vi "LVRT Serial Init.vi"(6 "stop bits (10: 1 bit)":u16(ring)=10 items=["1 bit"=10, "1.5 bits"=15, "2 bits"=20], 7 "Invert Polarity?":bool, 8 "error in (no error)":errorcluster, 9 "parity (0:none)":u16(ring) items=["None", "Odd", "Even", "Mark", "Space"], 10 "data bits (8)":u16=8 min=5 max=8 step=1, 11 "baud rate (9600)":u32=9600) -> (0 "error out":errorcluster, 3 "FPGA Main Reference Out":refnum<k20>)   [LabVIEW 2009]
uses:
  <vilib>/rvi/interface/nirviMethod/nirviMethod.xnode
  <vilib>/rvi/interface/nirviOpenFPGA/nirviOpenFPGA.xnode
  <vilib>/rvi/interface/nirviReadWriteControl/nirviReadWriteControl.xnode
  FPGA Main.vi
  FPGA Bitfiles/FPGA RS232.lvproj_FPGA Target_FPGA Main.vi.lvbit
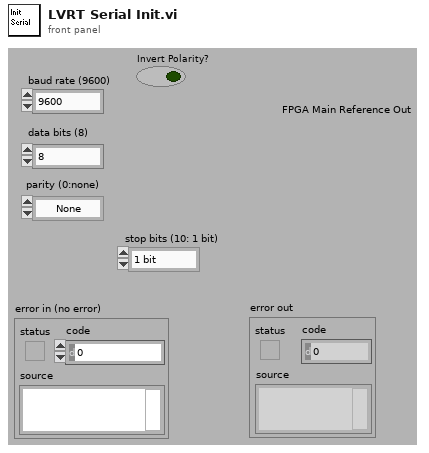
[diagram p1: front panel]
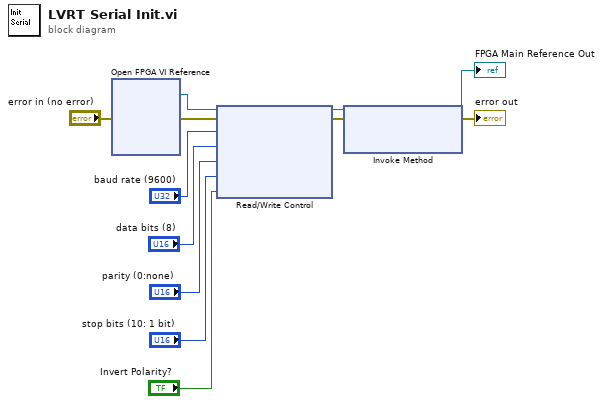
[diagram p0: block diagram]
diagram:
  n1 = xnode "Open FPGA VI Reference"("error in"="error in (no error)") -> ("FPGA VI Reference Out"=w12:refnum<k20>, "error out"=w11:errorcluster)  [unwired: 1 in]
  n2 = xnode "Read/Write Control"("FPGA VI Reference In"=w12, "error in"=w11, "baud rate (9600)"="baud rate (9600)", "data bits (8)"="data bits (8)", "parity (0:none)"="parity (0:none)", "stop bits (10: 1 bit)"="stop bits (10: 1 bit)", "Invert Polarity?"="Invert Polarity?") -> ("FPGA VI Reference Out"=w6:refnum<k20>, "error out"=w5:errorcluster)
  n3 = xnode "Invoke Method"("FPGA VI Reference In"=w6, "error in"=w5) -> ("FPGA VI Reference Out"=→"FPGA Main Reference Out":refnum<k20>, "error out"=→"error out":errorcluster)  [unwired: 1 out]
